vi "TagDB TagsChanged.vi"(8 "error in (no error)":errorcluster, 11 "DB Ref":T1) -> (0 "error in (no error) (dup)":errorcluster, 2 "item changed?":bool, 3 "DB Ref (dup)":T1)   [LabVIEW 2017, in "TagDB.lvlib"]
doc: "[Covers: REQ_API_DBITEMCHANGED]"
uses:
  TagDB.lvlib
  Typedef/TagDB.ctl
  Error/_[error50000]Invalid DB REF.vi
  DataAccess/TagDB Ref to DVR.vi
  Error/_Build Error Cluster.vi
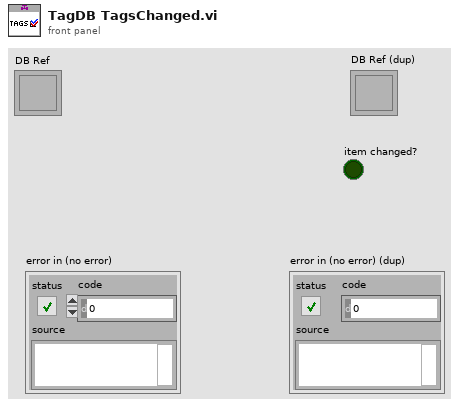
[diagram p1: front panel]
types:
  T1 = typedef "TagDB.lvlib/TagDB.ctl" = refnum<k1>
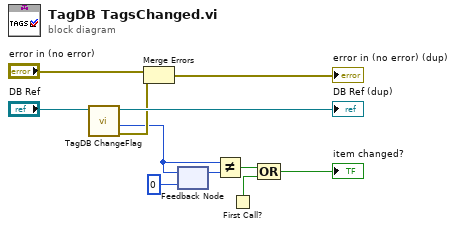
[diagram p0: block diagram]
diagram:
  n1 = call "TagDB ChangeFlag.vi"("DB Ref"="DB Ref") -> ("error in (no error) (dup)"=w7:errorcluster, "Item Change Timestamp"=w1:u64, "DB Ref (dup)"=→"DB Ref (dup)":T1)  [unwired: 7 in, 1 out]
  n2 = Merge Errors("error in (no error)", w7) -> (→"error in (no error) (dup)":errorcluster)
  n3 = feedback #1(u64 0 ("Global Change Timestamp")) -> (w2:u64)
  n4 = feedback-in #1(w1) -> ()
  n5 = Not Equal?(x=w1, y=w2) -> (x != y?=w5:bool)
  n6 = First Call?() -> (First Call?: T/F=w6:bool)
  n7 = Compound Arithmetic op=OR(w5, w6) -> (→"item changed?":bool)
